vi "intervalo.vi"(9 "incremento":dbl min=0.0, 10 "fin":dbl, 11 "inicio":dbl) -> (2 "Array":dbl[](array[numeric]))   [LabVIEW 2016]
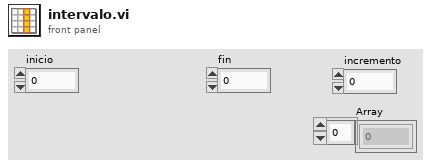
[diagram p1: front panel]
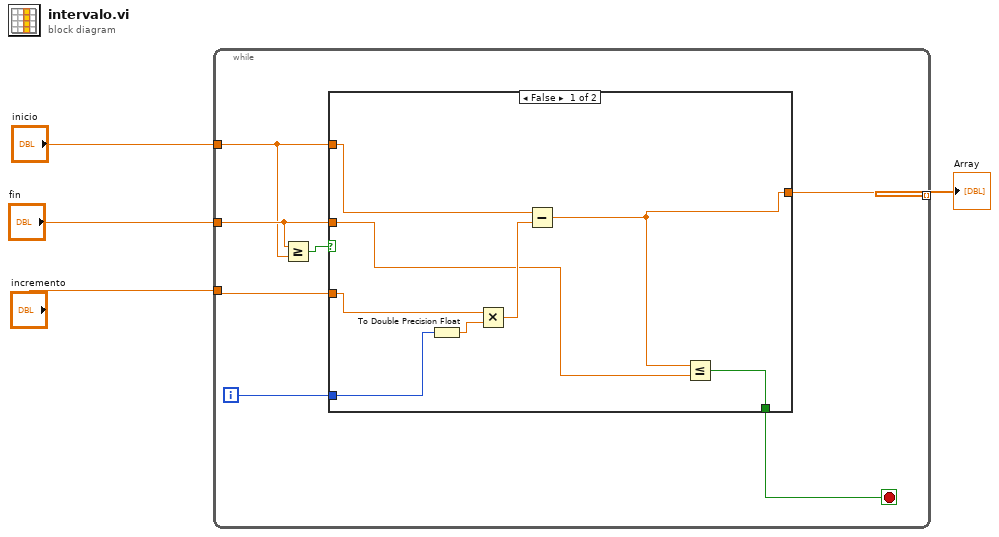
[diagram p0: block diagram]
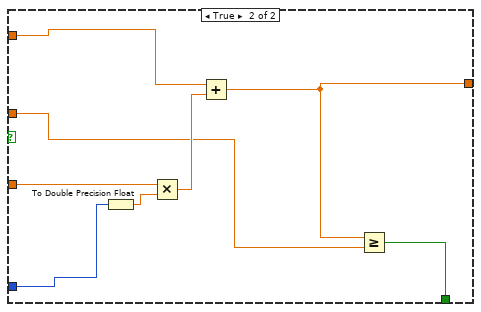
[diagram p2: hidden frame]
diagram:
  n1 = while {
    tunnel: "inicio" -> [w5]
    tunnel: "fin" -> [w6]
    tunnel: "incremento" -> [w11]
    tunnel: [w8] -> w1 mode=indexing
    i -> [w10]
    stop <- w9 stop-if-true
    n2 = Greater Or Equal?(x=w6, y=w5) -> (x >= y?=w7:bool)
    n3 = case shown="False" w7 {
      tunnel: w5 -> [w14 w27]
      tunnel: w11 -> [w16 w26]
      tunnel: w10 -> [w17 w24]
      tunnel: [w13 w22] -> w9
      tunnel: [w12 w21] -> w8
      tunnel: w6 -> [w15 w20]
      frame False {
        n4 = To Double Precision Float(number=w17) -> (double precision float=w19:dbl)
        n5 = Multiply(x=w16, y=w19) -> (x*y=w18:dbl)
        n6 = Subtract(x=w14, y=w18) -> (x-y=w12:dbl)
        n7 = Less Or Equal?(x=w12, y=w15) -> (x <= y?=w13:bool)
      }
      frame True {
        n8 = To Double Precision Float(number=w24) -> (double precision float=w25:dbl)
        n9 = Multiply(x=w26, y=w25) -> (x*y=w23:dbl)
        n10 = Add(x=w27, y=w23) -> (x+y=w21:dbl)
        n11 = Greater Or Equal?(x=w21, y=w20) -> (x >= y?=w22:bool)
      }
    }
  }
  "Array" <- w1
